vi "startIndex.vi"() -> (0 "Second":i32, 1 "startIndex":i32, 2 "minuteTOsecondStartIndex":i32, 3 "minuteStartIndex":i32)   [LabVIEW 2013]
doc: "the startIndex is how many seconds have past in this current half hour.\n\nthis subVI also returns the minute and the minute * 60 portion of each half hour for the purpose of calulating an initial index reference point."
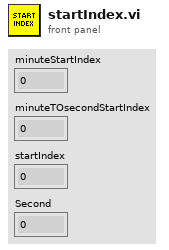
[diagram p1: front panel]
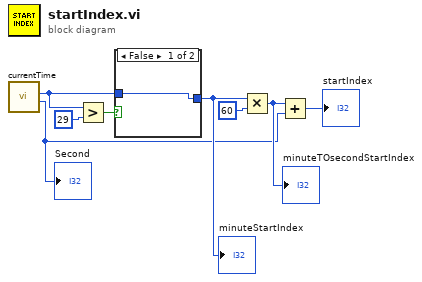
[diagram p0: block diagram]
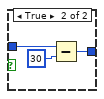
[diagram p2: hidden frame]
diagram:
  n1 = call "currentTime.vi"() -> ("Minute"=w8:i32, "Second"=w2:i32)  [unwired: 6 in, 1 out]
  "Second" <- w2
  n2 = Greater?(x=w8, y=29) -> (0:w7:bool)
  n3 = case shown="False" w7 {
    tunnel: w8 -> [w9 w12]
    tunnel: [w9 w10] -> w5
    frame False {
    }
    frame True {
      n4 = Subtract(x=w12, y=30) -> (x-y=w10:i32)
    }
  }
  "minuteStartIndex" <- w5
  n5 = Multiply(x=w5, y=60) -> (x*y=w3:i32)
  "minuteTOsecondStartIndex" <- w3
  n6 = Add(x=w3, y=w2) -> (x+y=→"startIndex":i32)
